vi "Z900_navX_Internal_Open.vi"(8 "error in":errorcluster, 11 "navX Device":T1={"Interface"={"Protocol"=enum."SERIAL", "Update Rate (4Hz-60Hz)"=4, "navX Open TypeDef"=variant}, "Notify Packet"=refnum, "Loop VI Refnum"=refnum, "Ready to Close Occurrence Refnum"=refnum} {"Interface"."Update Rate (4Hz-60Hz)" min=4 max=60 step=1}) -> (0 "error out":errorcluster, 2 "Interface TypeDefs":T3 {"I2CDevRef"."Device Address" format="%.0x"}, 3 "navX Device":T1={"Interface"={"Protocol"=enum."SERIAL", "Update Rate (4Hz-60Hz)"=4, "navX Open TypeDef"=variant}, "Notify Packet"=refnum, "Loop VI Refnum"=refnum, "Ready to Close Occurrence Refnum"=refnum} {"Interface"."Update Rate (4Hz-60Hz)" min=4 max=60 step=1})   [LabVIEW 2015, in "navX Library v2.lvlib"]
doc: "This navX VI handles opening the Serial/I2C/SPI reference for the navX.\nTHIS VI SHOULD NOT BE CALLED BY THE USER!"
uses:
  navX Library v2.lvlib
  TypeDefs/Z900_navX_DeviceTypeDef.ctl
  TypeDefs/Z900_navX_ProtocolTypeDef.ctl
  TypeDefs/Z900_navX_NotifyPacketTypeDef.ctl
  TypeDefs/Z900_navX_ActionTypeDef.ctl
  TypeDefs/Z900_navX_InterfaceTypeDef.ctl
  <vilib>/Rock Robotics/WPI/SerialPort/WPI_SerialPortRef.ctl
  <vilib>/Rock Robotics/WPI/I2C/WPI_I2CDevRef.ctl
  <vilib>/Rock Robotics/SystemInterfaces/i2clib/i2c_bus.ctl
  <vilib>/Rock Robotics/WPI/SPI/WPI_SPIDevRef.ctl
  <vilib>/Rock Robotics/SystemInterfaces/spilib/spi_bus.ctl
  TypeDefs/navX Open TypeDefs/Z900_navX_OpenTypeDef_I2C.ctl
  TypeDefs/navX Open TypeDefs/Z900_navX_OpenTypeDef_SPI.ctl
  TypeDefs/navX Open TypeDefs/Z900_navX_OpenTypeDef_Serial.ctl
  TypeDefs/Z900_navX_SerialStreamTypeDef.ctl
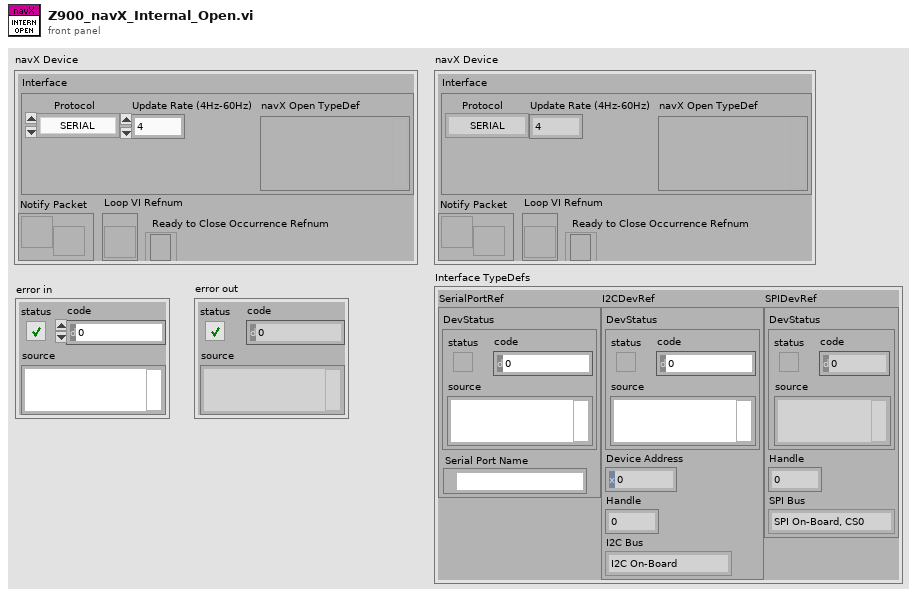
[diagram p1: front panel]
types:
  T1 = typedef "navX Library v2.lvlib/Z900_navX_DeviceTypeDef.ctl" = cluster{"Interface":cluster{"Protocol":T2, "Update Rate (4Hz-60Hz)":u8, "navX Open TypeDef":variant}, "Notify Packet":refnum<notifier>, "Loop VI Refnum":refnum<vi>, "Ready to Close Occurrence Refnum":refnum<k4>}
  T2 = typedef "navX Library v2.lvlib/Z900_navX_ProtocolTypeDef.ctl" = enum16{"SERIAL", "I2C", "SPI"}
  T3 = typedef "navX Library v2.lvlib/Z900_navX_InterfaceTypeDef.ctl" = cluster{"SerialPortRef":T4, "I2CDevRef":T5, "SPIDevRef":T7}
  T4 = typedef "WPI_SerialPortRef.ctl" = cluster{"DevStatus":errorcluster, "Serial Port Name":refnum<visa-resource-name>}
  T5 = typedef "WPI_I2CDevRef.ctl" = cluster{"DevStatus":errorcluster, "Device Address":u8, "Handle":i32, "I2C Bus":T6}
  T6 = typedef "i2c_bus.ctl" = enum16{"I2C On-Board", "I2C MXP", "Invalid"}
  T7 = typedef "WPI_SPIDevRef.ctl" = cluster{"DevStatus":errorcluster, "Handle":i32, "SPI Bus":T8}
  T8 = typedef "spi_bus.ctl" = enum16{"SPI On-Board, CS0", "SPI On-Board, CS1", "SPI On-Board, CS2", "SPI On-Board, CS3", "SPI MXP", "Invalid"}
  T9 = typedef "navX Library v2.lvlib/Z900_navX_OpenTypeDef_Serial.ctl" = cluster{"Serial Port":enum16{"Onboard RS-232", "MXP TTL", "USB"}, "Stream Type":T10}
  T10 = typedef "navX Library v2.lvlib/Z900_navX_SerialStreamTypeDef.ctl" = enum16{"YRPH", "Quaterinons", "Gyro/Raw", "AHRS", "AHRSAndPositioning"}
  T11 = typedef "navX Library v2.lvlib/Z900_navX_OpenTypeDef_I2C.ctl" = cluster{"I2C Bus":T6}
  T12 = typedef "navX Library v2.lvlib/Z900_navX_OpenTypeDef_SPI.ctl" = cluster{"SPI Bus":T8, "Clock Rate (Hz)":dbl}
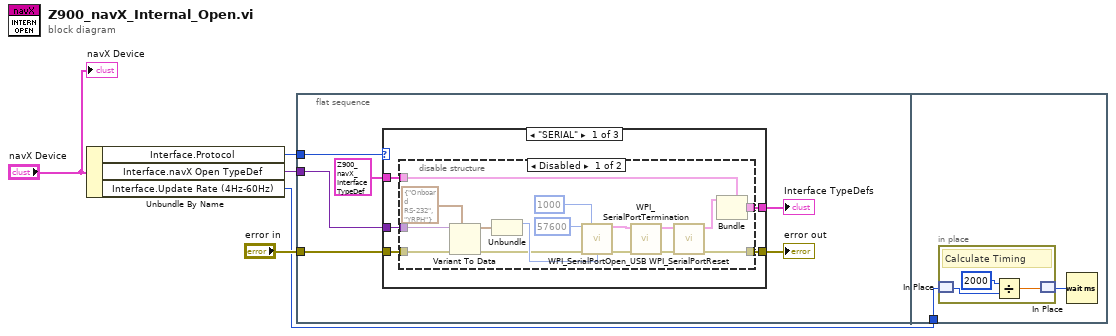
[diagram p0: block diagram]
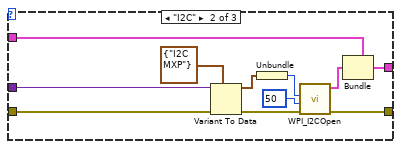
[diagram p3: hidden frame]
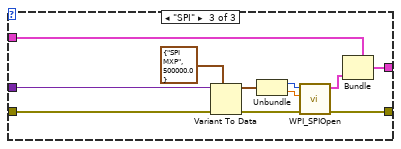
[diagram p4: hidden frame]
diagram:
  n1 = Unbundle By Name("navX Device") -> ("Interface.Protocol"=w5:T2, "Interface.navX Open TypeDef"=w4:variant, "Interface.Update Rate (4Hz-60Hz)"=w1:u8)
  n2 = flat-sequence {
    tunnel: w5 -> [w11]
    tunnel: w4 -> [w10]
    tunnel: "error in" -> [w8]
    tunnel: w1 -> [w55]
    frame #0 {
      n3 = case shown="\"SERIAL\"" w11 {
        tunnel: w10 -> [w16 w42 w53]
        tunnel: [w15 w38 w50] -> w9
        tunnel: w8 -> [w14 w36 w49]
        tunnel: T3 {"SerialPortRef"={"DevStatus"={"status"=FALSE, "code"=0, "source"=""}, "Serial Port Name"=""}, "I2CDevRef"={"DevStatus"={"status"=FALSE, "code"=0, "source"=""}, "Device Address"=0, "Handle"=0, "I2C Bus"=enum."I2C On-Board"}, "SPIDevRef"={"DevStatus"={"status"=FALSE, "code"=0, "source"=""}, "Handle"=0, "SPI Bus"=enum."SPI On-Board, CS0"}} ("Interface TypeDefs") -> [w12 w35 w47]
        tunnel: [w13 w34 w45] -> w6
        frame "SERIAL" {
          n4 = disable-structure shown="Disabled" {
            disable-tunnel: w16 -> [w32 _]
            disable-tunnel: [w24 _] -> w15
            disable-tunnel: w14 -> [w23 _]
            disable-tunnel: [w21 _] -> w13
            disable-tunnel: w12 -> [w20 _]
            frame Disabled {
              n5 = Variant To Data(error in=w23, type=T9 {"Serial Port"=enum."Onboard RS-232", "Stream Type"=enum."YRPH"} ("navX Serial Open"), Variant=w32) -> (data=w30:T9, error out=w22:errorcluster)
              n6 = Unbundle(w30) -> ("Serial Port"=w29:enum16{"Onboard RS-232", "MXP TTL", "USB"})  [unwired: 1 out]
              n7 = call "WPI_SerialPortOpen_USB.vi"("Baud Rate"=u32 57600, "Timeout Value (ms)"=u32 1000, "error in (no error)"=w22, "Serial Port"=w29) -> ("SerialPortRef"=w26:T4, "error out"=w25:errorcluster)  [unwired: 10 in]
              n8 = call <vilib>:"WPI_SerialPortTermination.vi"("error in (no error)"=w25, "SerialPortRef"=w26) -> ("error out"=w17:errorcluster, "SerialPortRef"=w18:T4)  [unwired: 8 in]
              n9 = call <vilib>:"WPI_SerialPortReset.vi"("error in (no error)"=w17, "SerialPortRef"=w18) -> ("error out"=w24:errorcluster, "SerialPortRef"=w19:T4)  [unwired: 8 in]
              n10 = Bundle(cluster=w20, "SerialPortRef"=w19) -> (w21:T3)  [unwired: 2 in]
            }
            frame Enabled {
            }
          }
        }
        frame "I2C" {
          n11 = Variant To Data(error in=w36, type=T11 {"I2C Bus"=enum."I2C MXP"} ("navX I2C Open"), Variant=w42) -> (data=w43:T11, error out=w37:errorcluster)
          n12 = Unbundle(w43) -> ("I2C Bus"=w40:T6)
          n13 = call <vilib>:"WPI_I2COpen.vi"("error in"=w37, "Device Address"=u8 50, "I2C Bus"=w40) -> ("error out"=w38:errorcluster, "I2CDevRef"=w33:T5)  [unwired: 7 in]
          n14 = Bundle(cluster=w35, "I2CDevRef"=w33) -> (w34:T3)  [unwired: 2 in]
        }
        frame "SPI" {
          n15 = Variant To Data(error in=w49, type=T12 {"SPI Bus"=enum."SPI MXP", "Clock Rate (Hz)"=500000.0} ("navX SPI Open"), Variant=w53) -> (data=w54:T12, error out=w48:errorcluster)
          n16 = Unbundle(w54) -> ("SPI Bus"=w51:T8, "Clock Rate (Hz)"=w44:dbl)
          n17 = call <vilib>:"WPI_SPIOpen.vi"("error in"=w48, "Clock Rate (Hz)"=w44, "SPI Bus"=w51) -> ("error out"=w50:errorcluster, "SPIDevRef"=w46:T7)  [unwired: 7 in]
          n18 = Bundle(cluster=w47, "SPIDevRef"=w46) -> (w45:T3)  [unwired: 2 in]
        }
      }
      "Interface TypeDefs" <- w6
      "error out" <- w9
    }
    frame #1 {
      n19 = in-place {
        # "Calculate Timing"
        n20 = in-place-match #1(w55) -> (w58:u8)
        n21 = Divide(x=2000, y=w58) -> (x/y=w57:dbl)
        n22 = in-place-match #1(w57) -> (w56:u8)
      }
      n23 = Wait (ms)(milliseconds to wait=w56) -> ()  [unwired: 1 out]
    }
  }
  "navX Device" <- "navX Device"
